vi "Split String.vi"(0 "string in":string, 5 "separator":string=" ") -> (4 "string array":string[](array[string]))   [LabVIEW 2015, in "LV String Utils v1.lvlib"]
doc: "Inspired by 'split' method of string class in Python."
uses:
  LV String Utils v1.lvlib
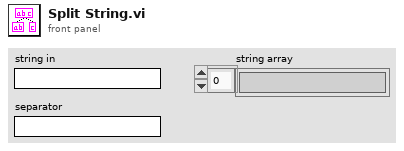
[diagram p1: front panel]
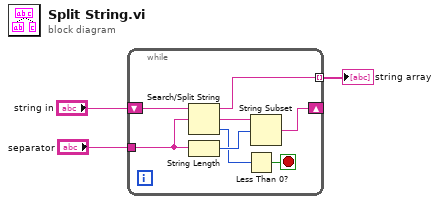
[diagram p0: block diagram]
diagram:
  n1 = while {
    shift-right: [w7] -> _
    shift-left: "string in" -> [w11]
    tunnel: [w10] -> w3 mode=indexing
    tunnel: "separator" -> [w4]
    stop <- w5 stop-if-true
    n2 = Search/Split String(string=w11, search string/char (-)=w4) -> (substring before match=w10:string, match + rest of string=w9:string, offset of match=w6:i32)  [unwired: 1 in]
    n3 = String Length(string=w4) -> (length=w8:i32)
    n4 = Less Than 0?(x=w6) -> (x < 0?=w5:bool)
    n5 = String Subset(string=w9, offset (0)=w8) -> (substring=w7:string)  [unwired: 1 in]
  }
  "string array" <- w3
